vi "步进获取点数.vi"(1 "步进":dbl, 2 "终止频率":dbl, 3 "起始频率":dbl) -> (0 "点数":i32)   [LabVIEW 2011]
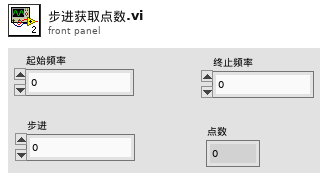
[diagram p1: front panel]
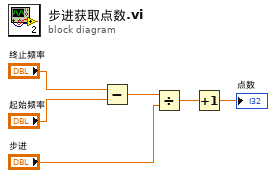
[diagram p0: block diagram]
diagram:
  n1 = Subtract(x="终止频率", y="起始频率") -> (x-y=w4:dbl)
  n2 = Divide(x=w4, y="步进") -> (x/y=w2:dbl)
  n3 = Increment(x=w2) -> (x+1=→"点数":dbl)
